vi "NmsBoxes.vi"(4 "nms_threshold":sgl, 5 "top_k":i32, 6 "score_threshold":sgl, 7 "eta":sgl=1.0, 8 "error in":errorcluster, 10 "scores":sgl[](array[numeric]), 11 "bboxes":T1[](array[typedef])) -> (0 "error out":errorcluster, 3 "indices":i32[](array[numeric]))   [LabVIEW 2020, in "OpenLvVision_OpenCv.lvlib"]
doc: "Performs non maximum suppression given boxes and corresponding scores."
uses:
  OpenLvVision_OpenCv.lvlib
  TypeDef/Rect2f.ctl
  Dlls/OlvOpenCvWrapper.dll
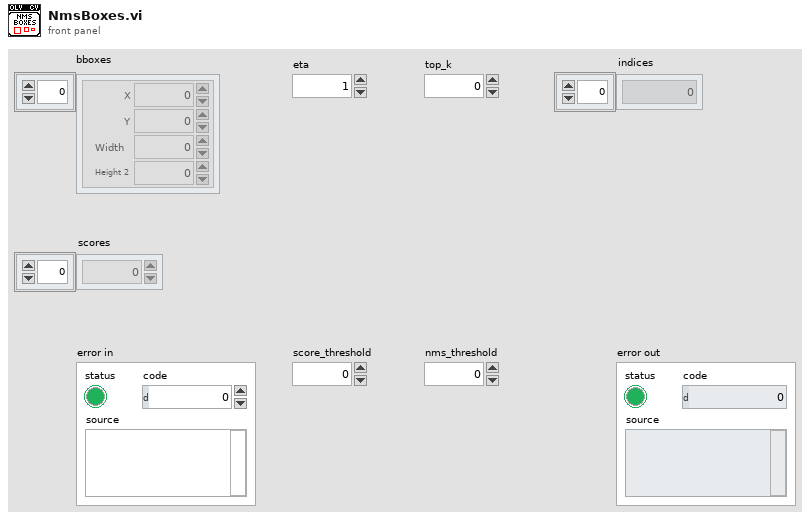
[diagram p1: front panel]
types:
  T1 = typedef "OpenLvVision_OpenCv.lvlib/Rect2f.ctl" = cluster{"X":sgl, "Y":sgl, "Width":sgl, "Height 2":sgl}
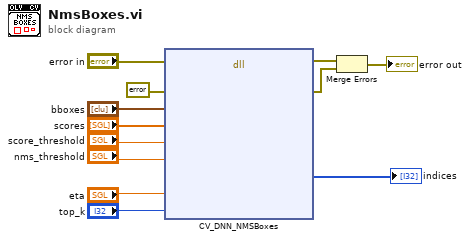
[diagram p0: block diagram]
diagram:
  n1 = dll-call lib="C:/Users/lukas/Downloads/OpenLvVision_OpenCv/SourceCode/LabView/OpenLvVision_OpenCv/Dlls/OlvOpenCvWrapper.dll" fn="CV_DNN_NMSBoxes"(error in="error in", "Error"=errorcluster {"status"=FALSE, "code"=0, "source"=""} ("error out"), "bboxesHandle"="bboxes", "scoresHandle"="scores", "scoreThreshold"="score_threshold", "nmsThreshold"="nms_threshold", "eta"="eta", "topK"="top_k") -> (error out=w12:errorcluster, "Error"=w10:errorcluster, "indicesHandle"=→"indices":i32[])  [unwired: 10 in, 1 out]
  n2 = Merge Errors(w12, w10) -> (→"error out":errorcluster)
